vi "Excel Formatting example.vi"() -> ()   [LabVIEW 2013]
panel:
  in  "DataFilePath":path
  in  "TemplatePath":path
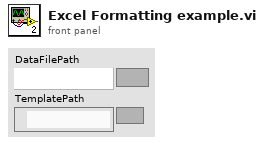
[diagram p1: front panel]
types:
  T1 = enum16{"", "xlEvaluateToError", "xlTextDate", "xlNumberAsText", "xlInconsistentFormula", "xlOmittedCells", "xlUnlockedFormulaCells", "xlEmptyCellReferences", "xlListDataValidation", "xlInconsistentListFormula"}
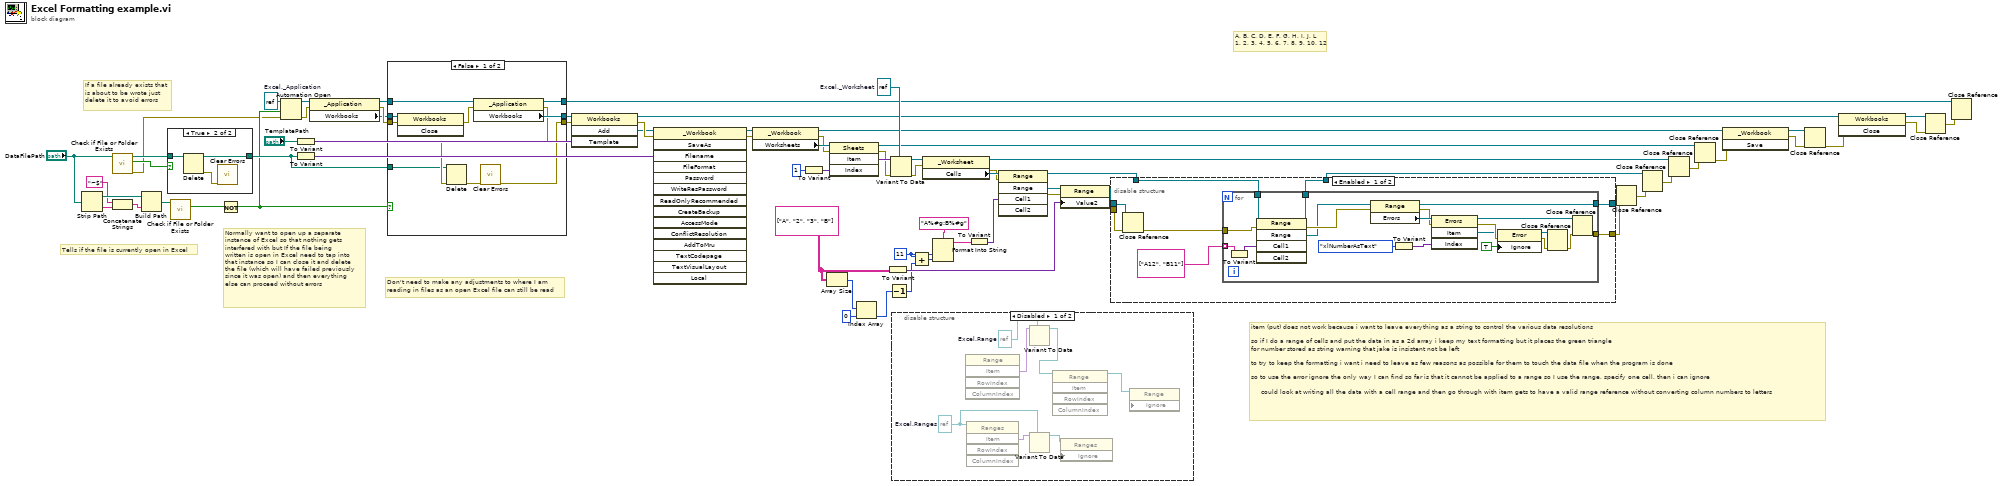
[diagram p0: block diagram]
diagram:
  w5 = string[][] [["A", "2"], ["3", "B"]]
  w9 = 11 ("index")
  w54 = refnum<k7> refnum  # Excel._Worksheet
  w44 = refnum<k7> refnum  # Excel._Application
  # "A, B, C, D, E, F, G, H, I, J, L\n1, 2, 3, 4, 5, 6, 7, 8, 9, 10, 12"
  # "item (put) does not work because i want to leave everything as a string to control the various data resolutions\n\nso if I do a range of cells and put the data in as a 2d array i keep my text formatting but it places the green triangle\nfor number stored as string warning that jake is insistent not be left\n\nto try to keep the formatting i want i need to leave as few reasons as possible for them to touch the data file when the program is done\n\nso to use the error ignore the only way I can find so far is that it cannot be applied to a range so I use the range, specify one cell, then i can ignore\n\n     could look at writing all the data with a cell range and then go through with item gets to have a valid range reference without converting column numbers to letters"
  # "Don't need to make any adjustments to where I am\nreading in files as an open Excel file can still be read"
  # "Normally want to open up a separate\ninstance of Excel so that nothing gets\ninterfered with but If the file being\nwritten is open in Excel need to tap into\nthat instance so I can close it and delete\nthe file (which will have failed previously\nsince it was open) and then everything\nelse can proceed without errors"
  # "Tells if the file is currently open in Excel"
  # "If a file already exists that\nis about to be wrote just\ndelete it to avoid errors"
  n1 = Strip Path(path="DataFilePath") -> (stripped path=w61:path, name=w60:string)
  n2 = call <vilib>:"Check if File or Folder Exists.vi"("path"="DataFilePath") -> ("error out"=w37:errorcluster, "file or folder exists?"=w56:bool)  [unwired: 8 in, 1 out]
  n3 = Concatenate Strings("~$" ("string"), w60) -> (w58:string)
  n4 = Build Path(base path=w61, name or relative path=w58) -> (appended path=w57:path)
  n5 = case shown="True" w56 {
    tunnel: "DataFilePath" -> [w72 w75]
    tunnel: [w72 w74] -> w70
    frame False {
    }
    frame True {
      n6 = Delete(path (use dialog)=w75) -> (deleted path=w74:path, error out=w73:errorcluster)  [unwired: 4 in, 1 out]
      n7 = call <vilib>:"Clear Errors.vi"("error in (no error)"=w73) -> ()  [unwired: 6 in, 1 out]
    }
  }
  n8 = call <vilib>:"Check if File or Folder Exists.vi"("path"=w57) -> ("file or folder exists?"=w63:bool)  [unwired: 8 in, 2 out]
  n9 = Not(x=w63) -> (.not. x?=w64:bool)
  n10 = Automation Open(error in (no error)=w37, Automation Refnum=w44, 9:w64) -> (Automation Refnum=w42:refnum<k7>, error out=w43:errorcluster)  [unwired: 1 in]
  n11 = To Variant(anything="TemplatePath") -> (Variant=w39:variant)
  n12 = To Variant(anything=w70) -> (Variant=w38:variant)
  n13 = property class="_Application"(reference=w42, error in=w43) -> (reference out=w69:refnum<k7>, error out=w66:errorcluster, "Workbooks"=w65:refnum<k7>)
  n14 = case shown="False" w64 {
    tunnel: w69 -> [w83 w88]
    tunnel: w65 -> [w85 w87]
    tunnel: w66 -> [w84 w86]
    tunnel: [w80 w87] -> w67
    tunnel: [w76 w86] -> w68
    tunnel: [w81 w88] -> w22
    tunnel: w70 -> [w77 _]
    frame False {
      n15 = invoke class="Workbooks" method="Close"(reference=w85, error in=w84) -> (error out=w82:errorcluster)  [unwired: 1 in, 2 out]
      n16 = property class="_Application"(reference=w83, error in=w82) -> (reference out=w81:refnum<k7>, error out=w78:errorcluster, "Workbooks"=w80:refnum<k7>)
      n17 = Delete(path (use dialog)=w77, error in=w78) -> (error out=w79:errorcluster)  [unwired: 3 in, 2 out]
      n18 = call <vilib>:"Clear Errors.vi"("error in (no error)"=w79) -> ("error out"=w76:errorcluster)  [unwired: 6 in]
    }
    frame True {
    }
  }
  n19 = invoke class="Workbooks" method="Add"(reference=w67, error in=w68, "Template"=w39) -> (reference out=w17:refnum<k7>, error out=w41:errorcluster, "Add"=w40:refnum<k7>)  [unwired: 1 in, 1 out]
  n20 = invoke class="_Workbook" method="SaveAs"(reference=w40, error in=w41, "Filename"=w38) -> (reference out=w53:refnum<k7>, error out=w55:errorcluster)  [unwired: 12 in, 13 out]
  n21 = property class="_Workbook"(reference=w53, error in=w55) -> (reference out=w16:refnum<k7>, error out=w50:errorcluster, "Worksheets"=w51:refnum<k7>)
  n22 = To Variant(anything=1) -> (Variant=w49:variant)
  n23 = Array Size(array=w5) -> (size(s)=w4:i32[])
  n24 = invoke class="Sheets" method="Item"(reference=w51, error in=w50, "Index"=w49) -> (reference out=w23:refnum<k7>, error out=w47:errorcluster, "Item"=w48:variant)  [unwired: 1 in, 1 out]
  n25 = Index Array(array=w4, index=0) -> (element=w2:i32)
  n26 = To Variant(anything=w5) -> (Variant=w33:variant)
  n27 = Decrement(x=w2) -> (x-1=w31:i32)
  n28 = Variant To Data(error in=w47, type=w54, Variant=w48) -> (data=w71:refnum<k7>, error out=w46:errorcluster)
  n29 = disable-structure shown="Disabled" {
    frame Disabled {
      w93 = refnum<k7> refnum  # Excel.Range
      w92 = refnum<k7> refnum  # Excel.Ranges
      n30 = invoke class="Range" method="Item"() -> ("Item"=w95:variant)  [unwired: 5 in, 4 out]
      n31 = invoke class="Ranges" method="Item"(reference=w92) -> ("Item"=w91:variant)  [unwired: 4 in, 4 out]
      n32 = Variant To Data(type=w93, Variant=w95) -> (data=w94:refnum<k7>)  [unwired: 1 in, 1 out]
      n33 = Variant To Data(type=w92, Variant=w91) -> (data=w90:refnum<k7>)  [unwired: 1 in, 1 out]
      n34 = invoke class="Range" method="Item"(reference=w94) -> (reference out=w89:refnum<k7>)  [unwired: 4 in, 4 out]
      n35 = property class="Ranges" props=["Ignore"](reference=w90) -> ()  [unwired: 2 in, 2 out]
      n36 = property class="Range" props=["Ignore"](reference=w89) -> ()  [unwired: 2 in, 2 out]
    }
    frame Enabled {
    }
  }
  n37 = Add(x=w9, y=w31) -> (x+y=w1:i32)
  n38 = property class="_Worksheet"(reference=w71, error in=w46) -> (reference out=w24:refnum<k7>, error out=w35:errorcluster, "Cells"=w36:refnum<k7>)
  n39 = Format Into String(format string="A%#g:B%#g", w9, w1) -> (resulting string=w32:string)  [unwired: 2 in, 1 out]
  n40 = To Variant(anything=w32) -> (Variant=w6:variant)
  n41 = invoke class="Range" method="Range"(reference=w36, error in=w35, "Cell1"=w6) -> (reference out=w8:refnum<k7>, error out=w34:errorcluster, "Range"=w29:refnum<k7>)  [unwired: 2 in, 2 out]
  n42 = property class="Range"(reference=w29, error in=w34, "Value2"=w33) -> (reference out=w28:refnum<k7>, error out=w26:errorcluster)
  n43 = disable-structure shown="Enabled" {
    disable-tunnel: w28 -> [w99 w125]
    disable-tunnel: [w103 w125] -> w27
    disable-tunnel: w26 -> [w98 w126]
    disable-tunnel: [w102 w126] -> w25
    disable-tunnel: w8 -> [w101 w124]
    disable-tunnel: [w100 w124] -> w7
    frame Enabled {
      n44 = Close Reference(reference=w99, error in (no error)=w98) -> (error out=w97:errorcluster)
      n45 = for {
        tunnel: [w123] -> w103
        tunnel: [w122] -> w102
        tunnel: w101 -> [w111]
        tunnel: [w110] -> w100
        tunnel: w97 -> [w109]
        tunnel: string[] ["A12", "B11"] -> [w106] mode=indexing
        n46 = To Variant(anything=w106) -> (Variant=w105:variant)
        n47 = invoke class="Range" method="Range"(reference=w111, error in=w109, "Cell1"=w105) -> (reference out=w110:refnum<k7>, error out=w108:errorcluster, "Range"=w107:refnum<k7>)  [unwired: 2 in, 2 out]
        n48 = property class="Range"(reference=w107, error in=w108) -> (reference out=w123:refnum<k7>, error out=w119:errorcluster, "Errors"=w121:refnum<k7>)
        n49 = To Variant(anything=T1."xlNumberAsText") -> (Variant=w113:variant)
        n50 = invoke class="Errors" method="Item"(reference=w121, error in=w119, "Index"=w113) -> (reference out=w115:refnum<k7>, error out=w118:errorcluster, "Item"=w104:refnum<k7>)  [unwired: 1 in, 1 out]
        n51 = property class="Error"(reference=w104, error in=w118, "Ignore"=TRUE) -> (reference out=w116:refnum<k7>, error out=w117:errorcluster)
        n52 = Close Reference(reference=w116, error in (no error)=w117) -> (error out=w114:errorcluster)
        n53 = Close Reference(reference=w115, error in (no error)=w114) -> (error out=w122:errorcluster)
      }
    }
    frame Disabled {
    }
  }
  n54 = Close Reference(reference=w27, error in (no error)=w25) -> (error out=w21:errorcluster)
  n55 = Close Reference(reference=w7, error in (no error)=w21) -> (error out=w20:errorcluster)
  n56 = Close Reference(reference=w24, error in (no error)=w20) -> (error out=w19:errorcluster)
  n57 = Close Reference(reference=w23, error in (no error)=w19) -> (error out=w11:errorcluster)
  n58 = invoke class="_Workbook" method="Save"(reference=w16, error in=w11) -> (reference out=w15:refnum<k7>, error out=w12:errorcluster)  [unwired: 1 in, 1 out]
  n59 = Close Reference(reference=w15, error in (no error)=w12) -> (error out=w10:errorcluster)
  n60 = invoke class="Workbooks" method="Close"(reference=w17, error in=w10) -> (reference out=w14:refnum<k7>, error out=w13:errorcluster)  [unwired: 1 in, 1 out]
  n61 = Close Reference(reference=w14, error in (no error)=w13) -> (error out=w18:errorcluster)
  n62 = Close Reference(reference=w22, error in (no error)=w18) -> ()  [unwired: 1 out]
